vi "4_belt_cam.vi"() -> ()   [LabVIEW 2022 SP3]
uses:
  <vilib>/userdefined/High Color/IMAQdx.ctl
  <vilib>/vision/Image Controls.llb/IMAQ Image.ctl
  <vilib>/vision/driver/NI_Vision_Acquisition_Software.lvlib
  <resource>/objmgr/imaqdx.rc
panel:
  in  "Tab Control":enum32{"Page 1", "Page 2", "Page 3"}(tab)
  in  "Next Button":bool
  out "Boolean 10":bool
  out "Boolean 9":bool
  out "Boolean 8":bool
  out "Boolean 7":bool
  out "Camera 4":T1(plugin-control)
  out "Camera 3":T1(plugin-control)
  out "Camera 2":T1(plugin-control)
  out "Camera 1":T1(plugin-control)
  in  "8":bool
  in  "7":bool
  in  "5":bool
  in  "1":bool
  in  "Refresh Button 3":bool caption="Refresh Button"
  in  "Refresh Button 2":bool caption="Refresh Button"
  in  "LOGIN STRING3":string
  in  "Previous Button":bool
  out "Exposure 4":dbl=150.0
  out "Exposure 3":dbl=150.0
  out "Exposure 2":dbl=150.0
  out "Exposure 1":dbl=150.0
  in  "Camera 4":bool=TRUE
  in  "Camera 3":bool=TRUE
  in  "Camera 2":bool=TRUE
  in  "Camera 1":bool=TRUE
  out "error out 13":errorcluster
  out "error out 12":errorcluster
  out "IMAQdx Session 6":T2
  in  "?":bool
  out "error out 15":errorcluster
  out "error out 14":errorcluster
  out "IMAQdx Session 7":T2
  in  "?":bool
  out "error out 17":errorcluster
  out "error out 16":errorcluster
  out "IMAQdx Session 8":T2
  in  "?":bool
  out "error out 21":errorcluster
  out "error out 20":errorcluster
  out "IMAQdx Session 10":T2
  in  "?":bool
  # "ENTER  PASSWORD"
  # "LOGIN"
  # "CANCEL"
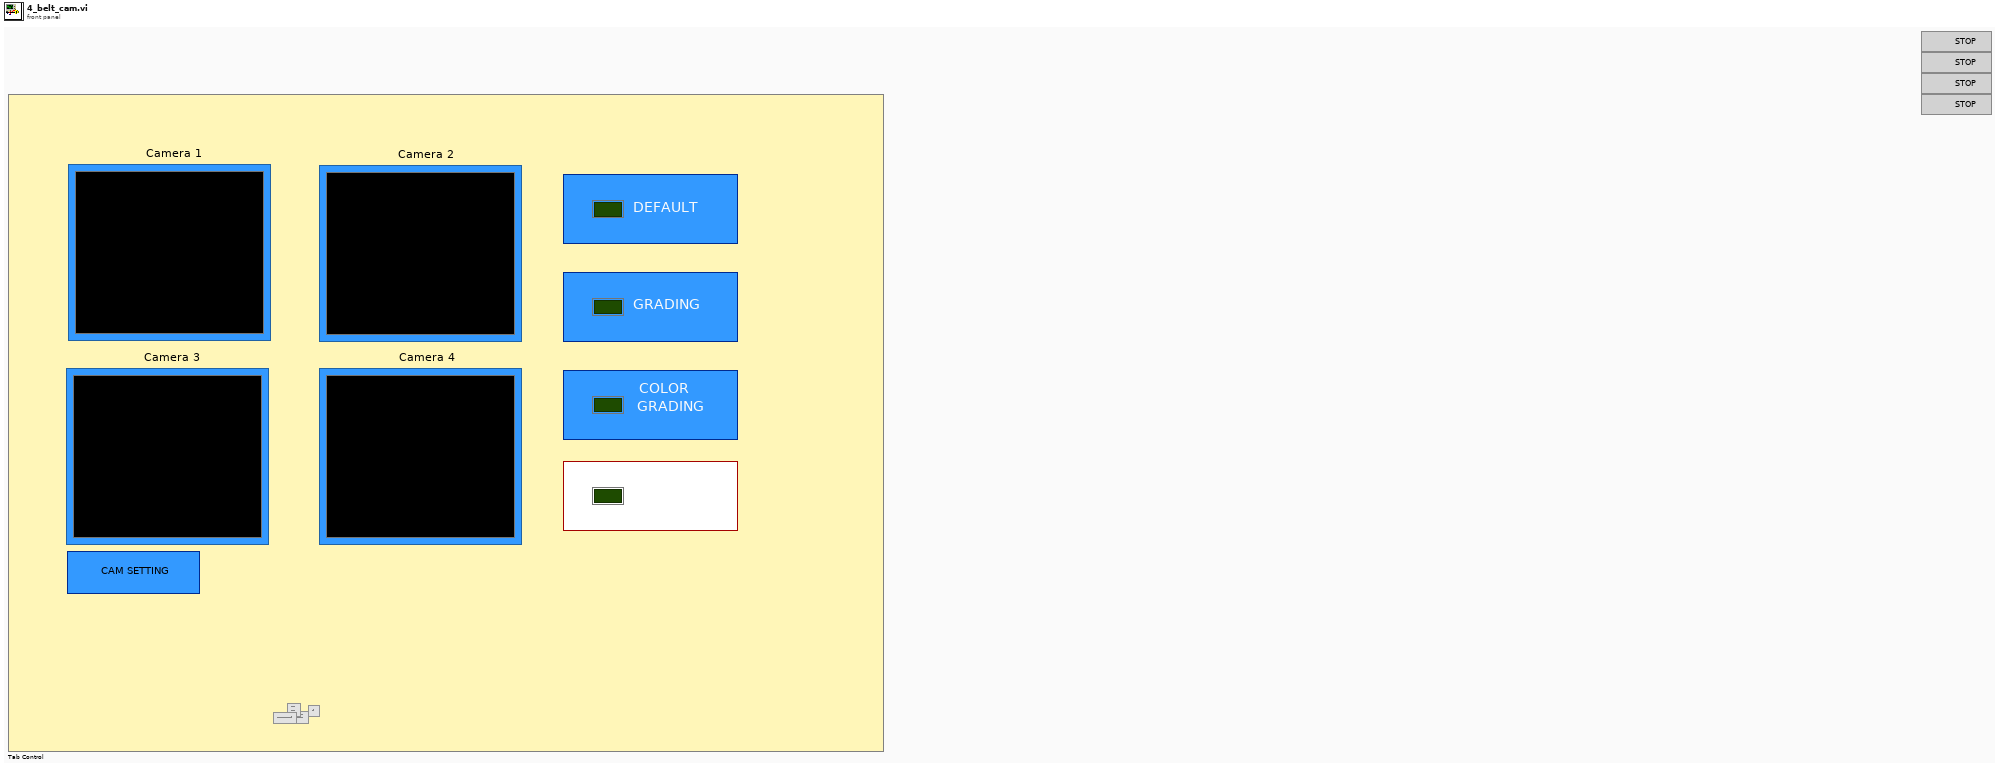
[diagram p1: front panel]
types:
  T1 = typedef "IMAQ Image.ctl" = refnum<image>
  T2 = typedef "IMAQdx.ctl" = refnum<k21>
  T3 = typedef "Image Type" = u32
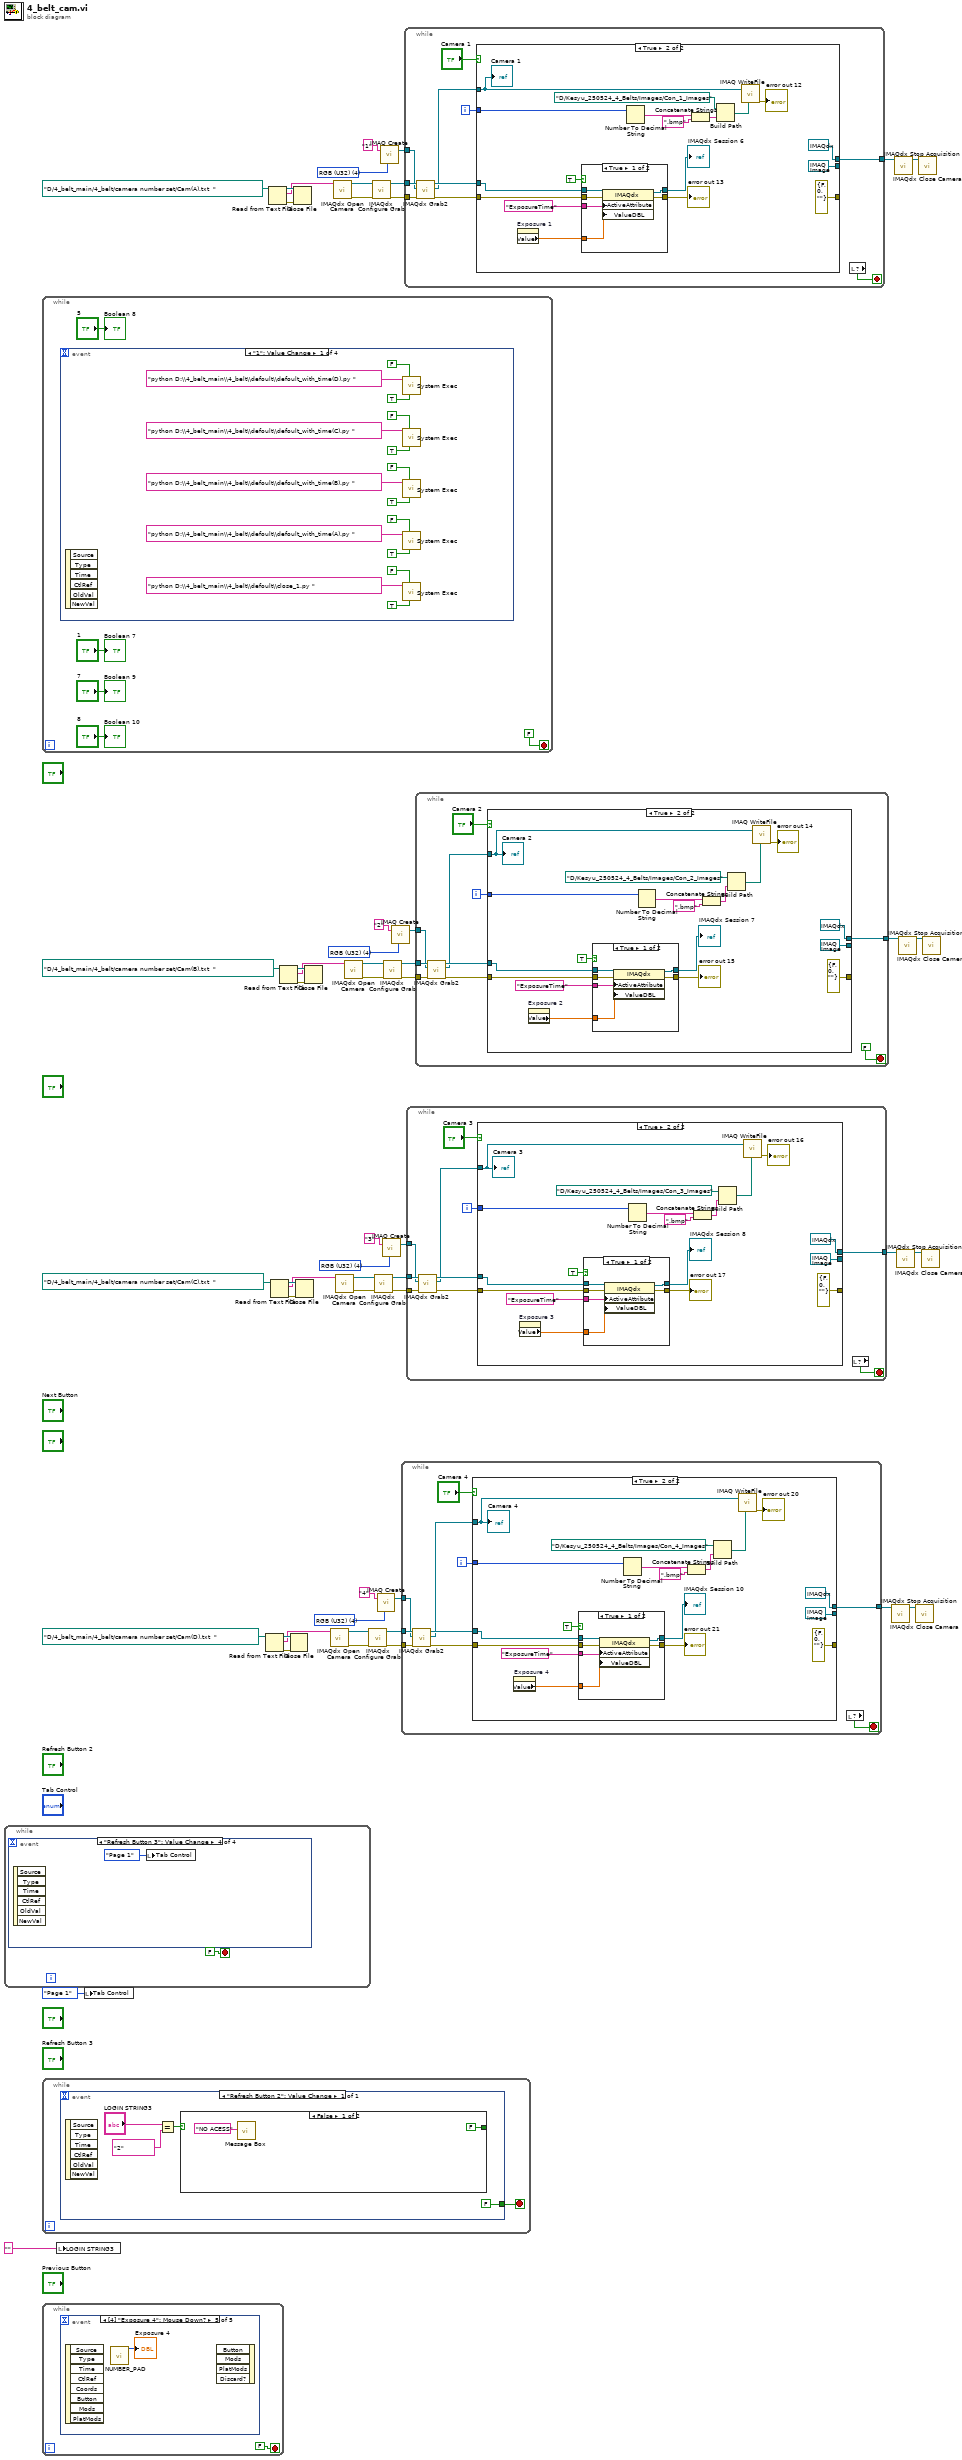
[diagram p0: block diagram]
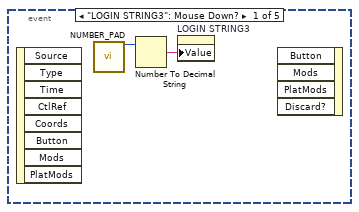
[diagram p2: hidden frame]
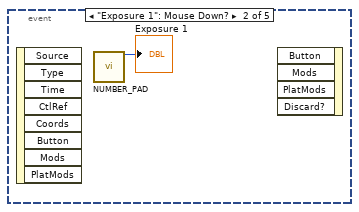
[diagram p3: hidden frame]
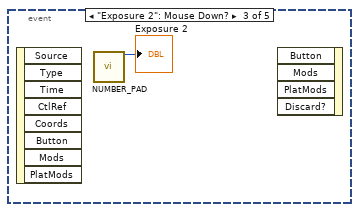
[diagram p4: hidden frame]
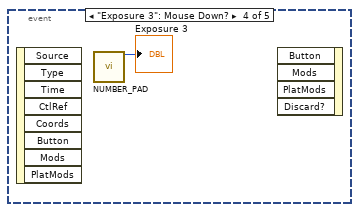
[diagram p5: hidden frame]
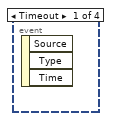
[diagram p6: hidden frame]
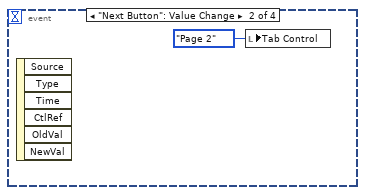
[diagram p7: hidden frame]
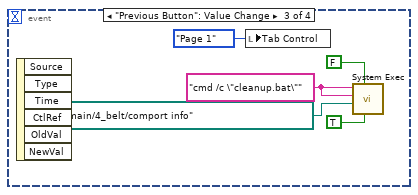
[diagram p8: hidden frame]
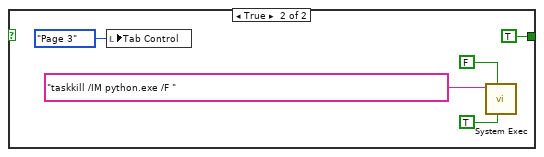
[diagram p9: hidden frame]
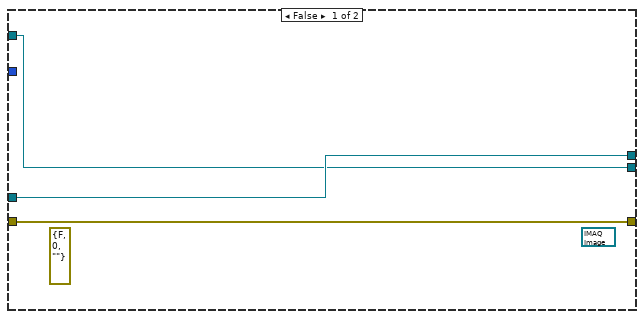
[diagram p10: hidden frame]
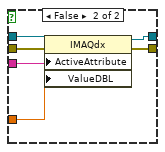
[diagram p11: hidden frame]
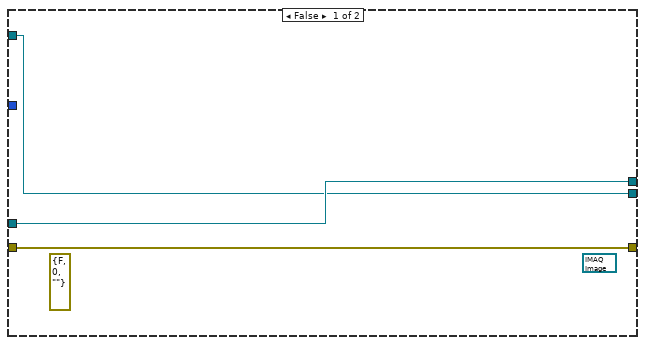
[diagram p12: hidden frame]
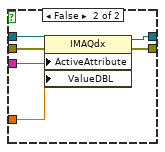
[diagram p13: hidden frame]
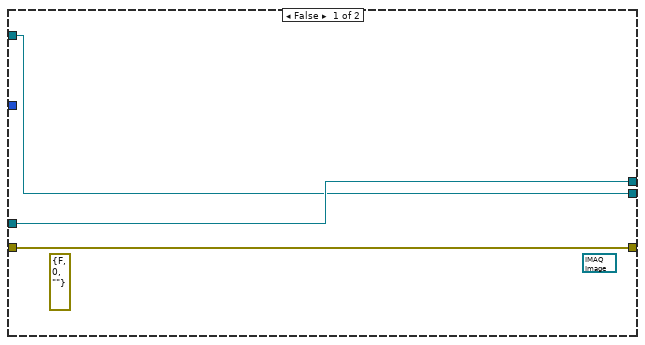
[diagram p14: hidden frame]
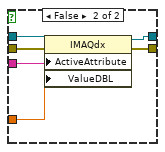
[diagram p15: hidden frame]
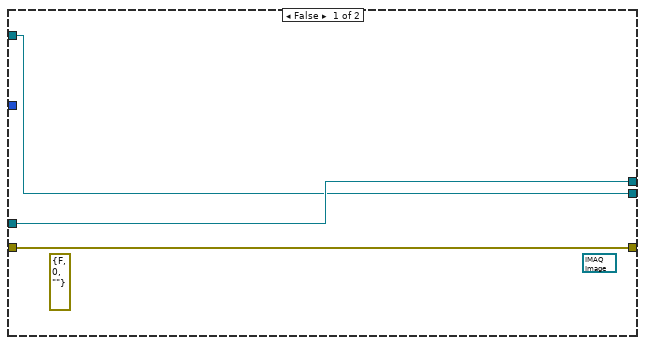
[diagram p16: hidden frame]
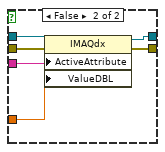
[diagram p17: hidden frame]
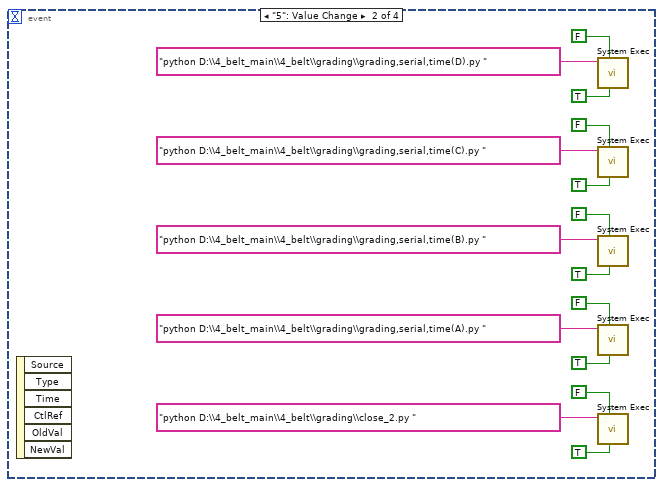
[diagram p18: hidden frame]
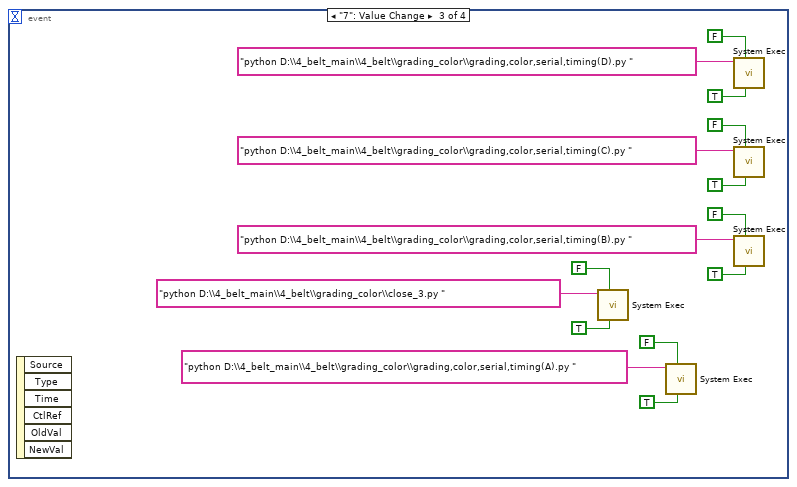
[diagram p19: hidden frame]
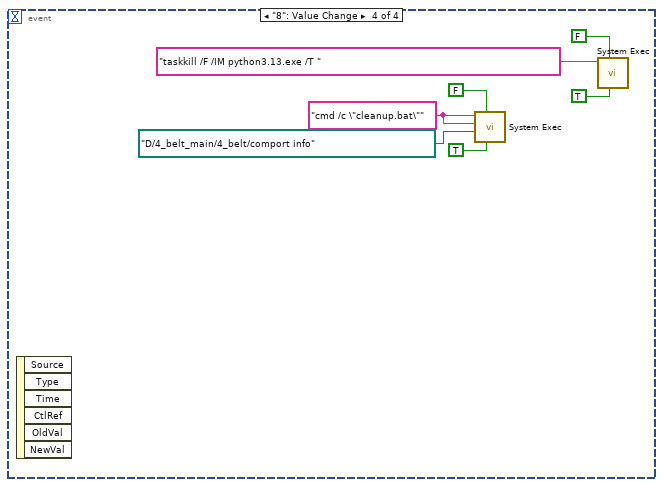
[diagram p20: hidden frame]
diagram:
  w23 = T3 4 items=["Grayscale (U8)", "Grayscale (I16)", "Grayscale (SGL)", "Complex (CSG)", "RGB (U32)", "HSL (U32)", "RGB (U64)", "Grayscale (U16)"] ("Image Type")
  w32 = T3 4 items=["Grayscale (U8)", "Grayscale (I16)", "Grayscale (SGL)", "Complex (CSG)", "RGB (U32)", "HSL (U32)", "RGB (U64)", "Grayscale (U16)"] ("Image Type")
  w41 = T3 4 items=["Grayscale (U8)", "Grayscale (I16)", "Grayscale (SGL)", "Complex (CSG)", "RGB (U32)", "HSL (U32)", "RGB (U64)", "Grayscale (U16)"] ("Image Type")
  w50 = T3 4 items=["Grayscale (U8)", "Grayscale (I16)", "Grayscale (SGL)", "Complex (CSG)", "RGB (U32)", "HSL (U32)", "RGB (U64)", "Grayscale (U16)"] ("Image Type")
  n1 = while {
    stop <- FALSE stop-if-true
    n2 = event shown="[3] \"Refresh Button 3\": Value Change" {
      selector: _ -> [_ _ _ _]
      dyn-events: _ -> [_ _ _ _]
      timeout: _ -> [_ _ _ _]
      event Timeout {
        n3 = event-data() -> ()  [unwired: 1 in, 3 out]
      }
      event "Next Button": Value Change {
        n4 = event-data() -> ()  [unwired: 1 in, 6 out]
        n5 = local write "Tab Control"(enum32{"Page 1", "Page 2", "Page 3"}."Page 2" ("Tab Control")) -> ()
      }
      event "Previous Button": Value Change {
        w58 = "cmd /c \"cleanup.bat\"" ("command line")
        n6 = event-data() -> ()  [unwired: 1 in, 6 out]
        n7 = local write "Tab Control"(enum32{"Page 1", "Page 2", "Page 3"}."Page 1" ("Tab Control")) -> ()
        n8 = call <vilib>:"System Exec.vi"("run minimized? (F)"=TRUE, "wait until completion? (T)"=FALSE, "working directory"=path "D:/4_belt_main/4_belt/comport info", "standard input"=w58, "command line"=w58) -> ()  [unwired: 3 in, 4 out]
      }
      event "Refresh Button 3": Value Change {
        n9 = event-data() -> ()  [unwired: 1 in, 6 out]
        n10 = local write "Tab Control"(enum32{"Page 1", "Page 2", "Page 3"}."Page 1" ("Tab Control")) -> ()
      }
    }
  }
  n11 = while {
    stop <- FALSE stop-if-true
    n12 = event shown="[0] \"1\": Value Change" {
      selector: _ -> [_ _ _ _]
      dyn-events: _ -> [_ _ _ _]
      timeout: _ -> [_ _ _ _]
      event "1": Value Change {
        n13 = event-data() -> ()  [unwired: 1 in, 6 out]
        n14 = call <vilib>:"System Exec.vi"("run minimized? (F)"=TRUE, "wait until completion? (T)"=FALSE, "command line"="python D:\\4_belt_main\\4_belt\\defoult\\defoult_with_time(D).py ") -> ()  [unwired: 5 in, 4 out]
        n15 = call <vilib>:"System Exec.vi"("run minimized? (F)"=TRUE, "wait until completion? (T)"=FALSE, "command line"="python D:\\4_belt_main\\4_belt\\defoult\\defoult_with_time(C).py ") -> ()  [unwired: 5 in, 4 out]
        n16 = call <vilib>:"System Exec.vi"("run minimized? (F)"=TRUE, "wait until completion? (T)"=FALSE, "command line"="python D:\\4_belt_main\\4_belt\\defoult\\defoult_with_time(B).py ") -> ()  [unwired: 5 in, 4 out]
        n17 = call <vilib>:"System Exec.vi"("run minimized? (F)"=TRUE, "wait until completion? (T)"=FALSE, "command line"="python D:\\4_belt_main\\4_belt\\defoult\\defoult_with_time(A).py ") -> ()  [unwired: 5 in, 4 out]
        n18 = call <vilib>:"System Exec.vi"("run minimized? (F)"=TRUE, "wait until completion? (T)"=FALSE, "command line"="python D:\\4_belt_main\\4_belt\\defoult\\close_1.py ") -> ()  [unwired: 5 in, 4 out]
      }
      event "5": Value Change {
        n19 = event-data() -> ()  [unwired: 1 in, 6 out]
        n20 = call <vilib>:"System Exec.vi"("run minimized? (F)"=TRUE, "wait until completion? (T)"=FALSE, "command line"="python D:\\4_belt_main\\4_belt\\grading\\grading,serial,time(D).py ") -> ()  [unwired: 5 in, 4 out]
        n21 = call <vilib>:"System Exec.vi"("run minimized? (F)"=TRUE, "wait until completion? (T)"=FALSE, "command line"="python D:\\4_belt_main\\4_belt\\grading\\grading,serial,time(C).py ") -> ()  [unwired: 5 in, 4 out]
        n22 = call <vilib>:"System Exec.vi"("run minimized? (F)"=TRUE, "wait until completion? (T)"=FALSE, "command line"="python D:\\4_belt_main\\4_belt\\grading\\grading,serial,time(B).py ") -> ()  [unwired: 5 in, 4 out]
        n23 = call <vilib>:"System Exec.vi"("run minimized? (F)"=TRUE, "wait until completion? (T)"=FALSE, "command line"="python D:\\4_belt_main\\4_belt\\grading\\grading,serial,time(A).py ") -> ()  [unwired: 5 in, 4 out]
        n24 = call <vilib>:"System Exec.vi"("run minimized? (F)"=TRUE, "wait until completion? (T)"=FALSE, "command line"="python D:\\4_belt_main\\4_belt\\grading\\close_2.py ") -> ()  [unwired: 5 in, 4 out]
      }
      event "7": Value Change {
        n25 = event-data() -> ()  [unwired: 1 in, 6 out]
        n26 = call <vilib>:"System Exec.vi"("run minimized? (F)"=TRUE, "wait until completion? (T)"=FALSE, "command line"="python D:\\4_belt_main\\4_belt\\grading_color\\close_3.py ") -> ()  [unwired: 5 in, 4 out]
        n27 = call <vilib>:"System Exec.vi"("run minimized? (F)"=TRUE, "wait until completion? (T)"=FALSE, "command line"="python D:\\4_belt_main\\4_belt\\grading_color\\grading,color,serial,timing(A).py ") -> ()  [unwired: 5 in, 4 out]
        n28 = call <vilib>:"System Exec.vi"("run minimized? (F)"=TRUE, "wait until completion? (T)"=FALSE, "command line"="python D:\\4_belt_main\\4_belt\\grading_color\\grading,color,serial,timing(D).py ") -> ()  [unwired: 5 in, 4 out]
        n29 = call <vilib>:"System Exec.vi"("run minimized? (F)"=TRUE, "wait until completion? (T)"=FALSE, "command line"="python D:\\4_belt_main\\4_belt\\grading_color\\grading,color,serial,timing(C).py ") -> ()  [unwired: 5 in, 4 out]
        n30 = call <vilib>:"System Exec.vi"("run minimized? (F)"=TRUE, "wait until completion? (T)"=FALSE, "command line"="python D:\\4_belt_main\\4_belt\\grading_color\\grading,color,serial,timing(B).py ") -> ()  [unwired: 5 in, 4 out]
      }
      event "8": Value Change {
        w114 = "cmd /c \"cleanup.bat\"" ("command line")
        n31 = event-data() -> ()  [unwired: 1 in, 6 out]
        n32 = call <vilib>:"System Exec.vi"("run minimized? (F)"=TRUE, "wait until completion? (T)"=FALSE, "working directory"=path "D:/4_belt_main/4_belt/comport info", "standard input"=w114, "command line"=w114) -> ()  [unwired: 3 in, 4 out]
        n33 = call <vilib>:"System Exec.vi"("run minimized? (F)"=TRUE, "wait until completion? (T)"=FALSE, "command line"="taskkill /F /IM python3.13.exe /T ") -> ()  [unwired: 5 in, 4 out]
      }
    }
    "Boolean 7" <- "1"
    "Boolean 8" <- "5"
    "Boolean 9" <- "7"
    "Boolean 10" <- "8"
  }
  n34 = while {
    stop <- w120 stop-if-true
    n35 = event shown="[0] \"Refresh Button 2\": Value Change" {
      selector: _ -> [_]
      dyn-events: _ -> [_]
      timeout: _ -> [_]
      tunnel: [FALSE] -> w120
      event "Refresh Button 2": Value Change {
        n36 = event-data() -> ()  [unwired: 1 in, 6 out]
        n37 = Equal?(x="LOGIN STRING3", y="2") -> (x = y?=w124:bool)
        n38 = case shown="False" w124 {
          tunnel: [FALSE TRUE] -> _
          frame False {
            n39 = call "Message Box.vi"("String"="NO ACESS") -> ()  [unwired: 9 in, 1 out]
          }
          frame True {
            n40 = local write "Tab Control"(enum32{"Page 1", "Page 2", "Page 3"}."Page 3" ("Tab Control")) -> ()
            n41 = call <vilib>:"System Exec.vi"("run minimized? (F)"=TRUE, "wait until completion? (T)"=FALSE, "command line"="taskkill /IM python.exe /F ") -> ()  [unwired: 5 in, 4 out]
          }
        }
      }
    }
  }
  n42 = while {
    stop <- FALSE stop-if-true
    n43 = event shown="[4] \"Exposure 4\": Mouse Down?" {
      selector: _ -> [_ _ _ _ _]
      dyn-events: _ -> [_ _ _ _ _]
      timeout: _ -> [_ _ _ _ _]
      event "LOGIN STRING3": Mouse Down? {
        n44 = event-data() -> ()  [unwired: 1 in, 8 out]
        n45 = call "NUMBER_PAD.vi"() -> ("number (out)"=w134:i32)  [unwired: 15 in]
        n46 = Number To Decimal String(number=w134) -> (decimal integer string=w133:string)  [unwired: 1 in]
        n47 = property on="LOGIN STRING3" class="Str"("Value"=w133) -> ()  [unwired: 2 in, 2 out]
        n48 = event-data() -> ()  [unwired: 5 in, 1 out]
      }
      event "Exposure 1": Mouse Down? {
        n49 = event-data() -> ()  [unwired: 1 in, 8 out]
        n50 = call "NUMBER_PAD.vi"() -> ("number (out)"=→"Exposure 1":i32)  [unwired: 15 in]
        n51 = event-data() -> ()  [unwired: 5 in, 1 out]
      }
      event "Exposure 2": Mouse Down? {
        n52 = event-data() -> ()  [unwired: 1 in, 8 out]
        n53 = call "NUMBER_PAD.vi"() -> ("number (out)"=→"Exposure 2":i32)  [unwired: 15 in]
        n54 = event-data() -> ()  [unwired: 5 in, 1 out]
      }
      event "Exposure 3": Mouse Down? {
        n55 = event-data() -> ()  [unwired: 1 in, 8 out]
        n56 = call "NUMBER_PAD.vi"() -> ("number (out)"=→"Exposure 3":i32)  [unwired: 15 in]
        n57 = event-data() -> ()  [unwired: 5 in, 1 out]
      }
      event "Exposure 4": Mouse Down? {
        n58 = event-data() -> ()  [unwired: 1 in, 8 out]
        n59 = call "NUMBER_PAD.vi"() -> ("number (out)"=→"Exposure 4":i32)  [unwired: 15 in]
        n60 = event-data() -> ()  [unwired: 5 in, 1 out]
      }
    }
  }
  n61 = local write "LOGIN STRING3"("" ("LOGIN STRING3")) -> ()
  n62 = local write "Tab Control"(enum32{"Page 1", "Page 2", "Page 3"}."Page 1" ("Tab Control")) -> ()
  n63 = Read from Text File(file (use dialog)=path "D:/4_belt_main/4_belt/camera number set/Cam(D).txt  ") -> (refnum out=w6:refnum<file>, text=w3:string, error out=w5:errorcluster)  [unwired: 3 in, 1 out]
  n64 = Read from Text File(file (use dialog)=path "D:/4_belt_main/4_belt/camera number set/Cam(A).txt  ") -> (refnum out=w18:refnum<file>, text=w15:string, error out=w17:errorcluster)  [unwired: 3 in, 1 out]
  n65 = Read from Text File(file (use dialog)=path "D:/4_belt_main/4_belt/camera number set/Cam(C).txt  ") -> (refnum out=w10:refnum<file>, text=w7:string, error out=w9:errorcluster)  [unwired: 3 in, 1 out]
  n66 = Read from Text File(file (use dialog)=path "D:/4_belt_main/4_belt/camera number set/Cam(B).txt  ") -> (refnum out=w14:refnum<file>, text=w11:string, error out=w13:errorcluster)  [unwired: 3 in, 1 out]
  n67 = Close File(refnum=w6, error in=w5) -> ()  [unwired: 2 out]
  n68 = Close File(refnum=w18, error in=w17) -> ()  [unwired: 2 out]
  n69 = Close File(refnum=w10, error in=w9) -> ()  [unwired: 2 out]
  n70 = Close File(refnum=w14, error in=w13) -> ()  [unwired: 2 out]
  n71 = call <vilib>:"IMAQdx Open Camera.vi"("Session In"=w3) -> ("error out"=w52:errorcluster, "Session Out"=w51:T2)  [unwired: 9 in]
  n72 = call <vilib>:"IMAQdx Open Camera.vi"("Session In"=w15) -> ("error out"=w25:errorcluster, "Session Out"=w24:T2)  [unwired: 9 in]
  n73 = call <vilib>:"IMAQdx Open Camera.vi"("Session In"=w7) -> ("error out"=w43:errorcluster, "Session Out"=w42:T2)  [unwired: 9 in]
  n74 = call <vilib>:"IMAQdx Open Camera.vi"("Session In"=w11) -> ("error out"=w34:errorcluster, "Session Out"=w33:T2)  [unwired: 9 in]
  n75 = call <vilib>:"IMAQdx Configure Grab.vi"("error in"=w52, "Session In"=w51) -> ("error out"=w53:errorcluster, "Session Out"=w54:T2)  [unwired: 8 in]
  n76 = call <vilib>:"IMAQdx Configure Grab.vi"("error in"=w25, "Session In"=w24) -> ("error out"=w26:errorcluster, "Session Out"=w27:T2)  [unwired: 8 in]
  n77 = call <vilib>:"IMAQdx Configure Grab.vi"("error in"=w43, "Session In"=w42) -> ("error out"=w44:errorcluster, "Session Out"=w45:T2)  [unwired: 8 in]
  n78 = call "IMAQ Create"("Image Name"="4", "Image Type"=w50) -> ("New Image"=w48:T1)  [unwired: 3 in, 1 out]
  n79 = call "IMAQ Create"("Image Name"="1", "Image Type"=w23) -> ("New Image"=w21:T1)  [unwired: 3 in, 1 out]
  n80 = call "IMAQ Create"("Image Name"="3", "Image Type"=w41) -> ("New Image"=w39:T1)  [unwired: 3 in, 1 out]
  n81 = call <vilib>:"IMAQdx Configure Grab.vi"("error in"=w34, "Session In"=w33) -> ("error out"=w35:errorcluster, "Session Out"=w36:T2)  [unwired: 8 in]
  n82 = call "IMAQ Create"("Image Name"="2", "Image Type"=w32) -> ("New Image"=w30:T1)  [unwired: 3 in, 1 out]
  n83 = while {
    tunnel: w48 -> [w143]
    tunnel: w53 -> [w145]
    tunnel: w54 -> [w144]
    tunnel: [w140] -> w47
    i -> [w148]
    stop <- w142 stop-if-true
    n84 = call <vilib>:"IMAQdx Grab2.vi"("error in"=w145, "Image In"=w143, "Session In"=w144) -> ("error out"=w147:errorcluster, "Image Out"=w141:T1, "Session Out"=w146:T2)  [unwired: 5 in, 1 out]
    n85 = case shown="True" "Camera 4" {
      tunnel: w148 -> [_ w165]
      tunnel: w147 -> [w149 w162]
      tunnel: w146 -> [w151 w160]
      tunnel: w141 -> [w150 w157]
      tunnel: [w151 T2 refnum ("Session Out")] -> w140
      tunnel: [w150 T1 refnum ("Image Out")] -> _
      tunnel: [w149 errorcluster {"status"=FALSE, "code"=0, "source"=""} ("error out")] -> _
      frame False {
        (unwired) errorcluster {"status"=FALSE, "code"=0, "source"=""} ("error out")
        (unwired) T1 refnum ("Image Out")
      }
      frame True {
        n86 = property on="Exposure 4" class="DigNum (strict)"() -> ("Value"=w152:dbl)  [unwired: 2 in, 2 out]
        n87 = case shown="True" TRUE {
          tunnel: w162 -> [w172 w181]
          tunnel: w160 -> [w174 w180]
          tunnel: [w175 w179] -> w161
          tunnel: [w173 w178] -> w159
          tunnel: "ExposureTime" ("ActiveAttribute") -> [w171 w177]
          tunnel: w152 -> [w170 w176]
          frame True {
            n88 = property class="IMAQdx"(reference=w174, error in=w172, "ActiveAttribute"=w171, "ValueDBL"=w170) -> (reference out=w175:T2, error out=w173:errorcluster)
          }
          frame False {
            n89 = property class="IMAQdx"(reference=w180, error in=w181, "ActiveAttribute"=w177, "ValueDBL"=w176) -> (reference out=w179:T2, error out=w178:errorcluster)
          }
        }
        "error out 21" <- w159
        "IMAQdx Session 10" <- w161
        n90 = Number To Decimal String(number=w165) -> (decimal integer string=w166:string)  [unwired: 1 in]
        n91 = Concatenate Strings(w166, ".bmp" ("pattern (all files)")) -> (w167:string)
        n92 = Build Path(base path=path "D:/Kesyu_250524_4_Belts/Images/Con_4_Images", name or relative path=w167) -> (appended path=w168:path)
        n93 = call "IMAQ WriteFile"("File Path"=w168, "Image"=w157) -> ("error out"=→"error out 20":errorcluster)  [unwired: 3 in, 3 out]
        "Camera 4" <- w157
      }
    }
    n94 = local read item#4() -> (w142:bool)
  }
  n95 = while {
    tunnel: w21 -> [w186]
    tunnel: w26 -> [w188]
    tunnel: w27 -> [w187]
    tunnel: [w183] -> w20
    i -> [w191]
    stop <- w185 stop-if-true
    n96 = call <vilib>:"IMAQdx Grab2.vi"("error in"=w188, "Image In"=w186, "Session In"=w187) -> ("error out"=w190:errorcluster, "Image Out"=w184:T1, "Session Out"=w189:T2)  [unwired: 5 in, 1 out]
    n97 = case shown="True" "Camera 1" {
      tunnel: w191 -> [_ w208]
      tunnel: w190 -> [w192 w205]
      tunnel: w189 -> [w194 w203]
      tunnel: w184 -> [w193 w200]
      tunnel: [w194 T2 refnum ("Session Out")] -> w183
      tunnel: [w193 T1 refnum ("Image Out")] -> _
      tunnel: [w192 errorcluster {"status"=FALSE, "code"=0, "source"=""} ("error out")] -> _
      frame False {
        (unwired) errorcluster {"status"=FALSE, "code"=0, "source"=""} ("error out")
        (unwired) T1 refnum ("Image Out")
      }
      frame True {
        n98 = property on="Exposure 1" class="DigNum (strict)"() -> ("Value"=w195:dbl)  [unwired: 2 in, 2 out]
        n99 = case shown="True" TRUE {
          tunnel: w205 -> [w215 w224]
          tunnel: w203 -> [w217 w223]
          tunnel: [w218 w222] -> w204
          tunnel: [w216 w221] -> w202
          tunnel: "ExposureTime" ("ActiveAttribute") -> [w214 w220]
          tunnel: w195 -> [w213 w219]
          frame True {
            n100 = property class="IMAQdx"(reference=w217, error in=w215, "ActiveAttribute"=w214, "ValueDBL"=w213) -> (reference out=w218:T2, error out=w216:errorcluster)
          }
          frame False {
            n101 = property class="IMAQdx"(reference=w223, error in=w224, "ActiveAttribute"=w220, "ValueDBL"=w219) -> (reference out=w222:T2, error out=w221:errorcluster)
          }
        }
        "error out 13" <- w202
        "IMAQdx Session 6" <- w204
        n102 = Number To Decimal String(number=w208) -> (decimal integer string=w209:string)  [unwired: 1 in]
        n103 = Concatenate Strings(w209, ".bmp" ("pattern (all files)")) -> (w210:string)
        n104 = Build Path(base path=path "D:/Kesyu_250524_4_Belts/Images/Con_1_Images", name or relative path=w210) -> (appended path=w211:path)
        n105 = call "IMAQ WriteFile"("File Path"=w211, "Image"=w200) -> ("error out"=→"error out 12":errorcluster)  [unwired: 3 in, 3 out]
        "Camera 1" <- w200
      }
    }
    n106 = local read item#22() -> (w185:bool)
  }
  n107 = while {
    tunnel: w39 -> [w229]
    tunnel: w44 -> [w231]
    tunnel: w45 -> [w230]
    tunnel: [w226] -> w38
    i -> [w234]
    stop <- w228 stop-if-true
    n108 = call <vilib>:"IMAQdx Grab2.vi"("error in"=w231, "Image In"=w229, "Session In"=w230) -> ("error out"=w233:errorcluster, "Image Out"=w227:T1, "Session Out"=w232:T2)  [unwired: 5 in, 1 out]
    n109 = case shown="True" "Camera 3" {
      tunnel: w234 -> [_ w251]
      tunnel: w233 -> [w235 w248]
      tunnel: w232 -> [w237 w246]
      tunnel: w227 -> [w236 w243]
      tunnel: [w237 T2 refnum ("Session Out")] -> w226
      tunnel: [w236 T1 refnum ("Image Out")] -> _
      tunnel: [w235 errorcluster {"status"=FALSE, "code"=0, "source"=""} ("error out")] -> _
      frame False {
        (unwired) errorcluster {"status"=FALSE, "code"=0, "source"=""} ("error out")
        (unwired) T1 refnum ("Image Out")
      }
      frame True {
        n110 = property on="Exposure 3" class="DigNum (strict)"() -> ("Value"=w238:dbl)  [unwired: 2 in, 2 out]
        n111 = case shown="True" TRUE {
          tunnel: w248 -> [w258 w267]
          tunnel: w246 -> [w260 w266]
          tunnel: [w261 w265] -> w247
          tunnel: [w259 w264] -> w245
          tunnel: "ExposureTime" ("ActiveAttribute") -> [w257 w263]
          tunnel: w238 -> [w256 w262]
          frame True {
            n112 = property class="IMAQdx"(reference=w260, error in=w258, "ActiveAttribute"=w257, "ValueDBL"=w256) -> (reference out=w261:T2, error out=w259:errorcluster)
          }
          frame False {
            n113 = property class="IMAQdx"(reference=w266, error in=w267, "ActiveAttribute"=w263, "ValueDBL"=w262) -> (reference out=w265:T2, error out=w264:errorcluster)
          }
        }
        "error out 17" <- w245
        "IMAQdx Session 8" <- w247
        n114 = Number To Decimal String(number=w251) -> (decimal integer string=w252:string)  [unwired: 1 in]
        n115 = Concatenate Strings(w252, ".bmp" ("pattern (all files)")) -> (w253:string)
        n116 = Build Path(base path=path "D:/Kesyu_250524_4_Belts/Images/Con_3_Images", name or relative path=w253) -> (appended path=w254:path)
        n117 = call "IMAQ WriteFile"("File Path"=w254, "Image"=w243) -> ("error out"=→"error out 16":errorcluster)  [unwired: 3 in, 3 out]
        "Camera 3" <- w243
      }
    }
    n118 = local read item#10() -> (w228:bool)
  }
  n119 = while {
    tunnel: w30 -> [w272]
    tunnel: w35 -> [w274]
    tunnel: w36 -> [w273]
    tunnel: [w269] -> w29
    i -> [w277]
    stop <- FALSE stop-if-true
    n120 = call <vilib>:"IMAQdx Grab2.vi"("error in"=w274, "Image In"=w272, "Session In"=w273) -> ("error out"=w276:errorcluster, "Image Out"=w270:T1, "Session Out"=w275:T2)  [unwired: 5 in, 1 out]
    n121 = case shown="True" "Camera 2" {
      tunnel: w277 -> [_ w294]
      tunnel: w276 -> [w278 w291]
      tunnel: w275 -> [w280 w289]
      tunnel: w270 -> [w279 w286]
      tunnel: [w280 T2 refnum ("Session Out")] -> w269
      tunnel: [w279 T1 refnum ("Image Out")] -> _
      tunnel: [w278 errorcluster {"status"=FALSE, "code"=0, "source"=""} ("error out")] -> _
      frame False {
        (unwired) errorcluster {"status"=FALSE, "code"=0, "source"=""} ("error out")
        (unwired) T1 refnum ("Image Out")
      }
      frame True {
        n122 = property on="Exposure 2" class="DigNum (strict)"() -> ("Value"=w281:dbl)  [unwired: 2 in, 2 out]
        n123 = case shown="True" TRUE {
          tunnel: w291 -> [w301 w310]
          tunnel: w289 -> [w303 w309]
          tunnel: [w304 w308] -> w290
          tunnel: [w302 w307] -> w288
          tunnel: "ExposureTime" ("ActiveAttribute") -> [w300 w306]
          tunnel: w281 -> [w299 w305]
          frame True {
            n124 = property class="IMAQdx"(reference=w303, error in=w301, "ActiveAttribute"=w300, "ValueDBL"=w299) -> (reference out=w304:T2, error out=w302:errorcluster)
          }
          frame False {
            n125 = property class="IMAQdx"(reference=w309, error in=w310, "ActiveAttribute"=w306, "ValueDBL"=w305) -> (reference out=w308:T2, error out=w307:errorcluster)
          }
        }
        "error out 15" <- w288
        "IMAQdx Session 7" <- w290
        n126 = Number To Decimal String(number=w294) -> (decimal integer string=w295:string)  [unwired: 1 in]
        n127 = Concatenate Strings(w295, ".bmp" ("pattern (all files)")) -> (w296:string)
        n128 = Build Path(base path=path "D:/Kesyu_250524_4_Belts/Images/Con_2_Images", name or relative path=w296) -> (appended path=w297:path)
        n129 = call "IMAQ WriteFile"("File Path"=w297, "Image"=w286) -> ("error out"=→"error out 14":errorcluster)  [unwired: 3 in, 3 out]
        "Camera 2" <- w286
      }
    }
  }
  n130 = call <vilib>:"IMAQdx Stop Acquisition.vi"("Session In"=w47) -> ("Session Out"=w46:T2)  [unwired: 9 in, 1 out]
  n131 = call <vilib>:"IMAQdx Stop Acquisition.vi"("Session In"=w20) -> ("Session Out"=w19:T2)  [unwired: 9 in, 1 out]
  n132 = call <vilib>:"IMAQdx Stop Acquisition.vi"("Session In"=w38) -> ("Session Out"=w37:T2)  [unwired: 9 in, 1 out]
  n133 = call <vilib>:"IMAQdx Stop Acquisition.vi"("Session In"=w29) -> ("Session Out"=w28:T2)  [unwired: 9 in, 1 out]
  n134 = call <vilib>:"IMAQdx Close Camera.vi"("Session In"=w46) -> ()  [unwired: 10 in, 1 out]
  n135 = call <vilib>:"IMAQdx Close Camera.vi"("Session In"=w19) -> ()  [unwired: 10 in, 1 out]
  n136 = call <vilib>:"IMAQdx Close Camera.vi"("Session In"=w37) -> ()  [unwired: 10 in, 1 out]
  n137 = call <vilib>:"IMAQdx Close Camera.vi"("Session In"=w28) -> ()  [unwired: 10 in, 1 out]
